vi "Check Bounds (Buffer).vi"(5 "source vi name":string, 7 "buffer size":u64 format="%d bytes", 8 "error in (no error)":errorcluster, 9 "offset (0)":u64 format="%d bytes", 10 "size to move":u64 format="%d bytes", 11 "Pointer in":refnum<class "Pointer.lvclass">) -> (0 "error out":errorcluster, 1 "offset":u64 format="%d bytes", 2 "size to move":u64 format="%d bytes", 3 "Pointer out":refnum<class "Pointer.lvclass">)   [LabVIEW 2017, in "Memory Manager.lvlib" / "Pointer.lvclass"]
uses:
  Pointer.lvclass
  Buffer Underflow.vi
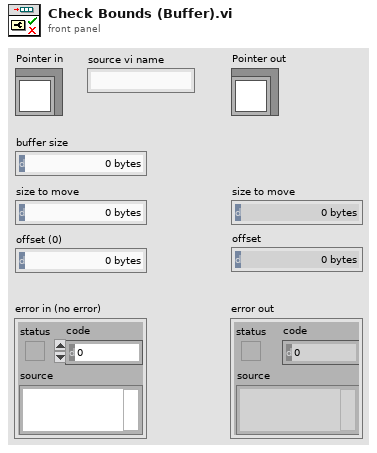
[diagram p1: front panel]
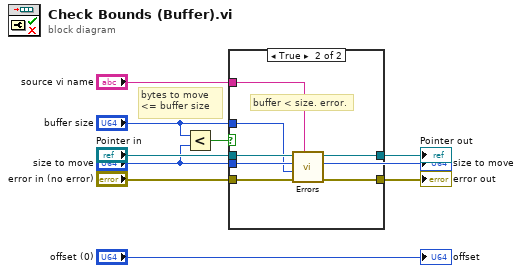
[diagram p0: block diagram]
diagram:
  # "bytes to move <= buffer size"
  n1 = Less?(x="buffer size", y="size to move") -> (x < y?=w6:bool)
  n2 = case shown="True" w6 {
    tunnel: "source vi name" -> [_ w12]
    tunnel: "buffer size" -> [_ w16]
    tunnel: "Pointer in" -> [w11 w18]
    tunnel: "size to move" -> [_ w17]
    tunnel: "error in (no error)" -> [w10 w15]
    tunnel: [w11 w14] -> w4
    tunnel: [w10 w13] -> w3
    frame False {
      # "buffer size is large enough. proceed."
    }
    frame True {
      # "buffer < size. error."
      n3 = call-poly "Errors.vi"("error source vi name"=w12, "error in (no error)"=w15, "actual buffer size"=w16, "required buffer size"=w17, "Pointer in"=w18) -> ("error out"=w13:errorcluster, "Pointer out"=w14:refnum<class "Pointer.lvclass">)  [unwired: 5 in]
    }
  }
  "error out" <- w3
  "Pointer out" <- w4
  "size to move" <- "size to move"
  "offset" <- "offset (0)"
